vi "Get Unix Timestamp.vi"() -> (2 "Unix Timestamp":u64)   [LabVIEW 2011, in "i3-oauth.lvlib"]
doc: "Gets the Current Time in Unix Timestamp format."
uses:
  i3-oauth.lvlib
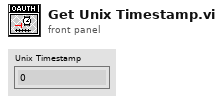
[diagram p1: front panel]
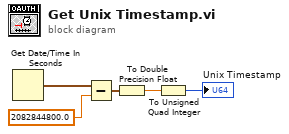
[diagram p0: block diagram]
diagram:
  n1 = Get Date/Time In Seconds() -> (seconds since 1Jan1904=w2:timestamp)
  n2 = Subtract(x=w2, y=2082844800.0) -> (x-y=w4:timestamp)
  n3 = To Double Precision Float(number=w4) -> (double precision float=w5:dbl)
  n4 = To Unsigned Quad Integer(1:w5) -> (0:→"Unix Timestamp":u64)
